vi "TestFastLocalizeCPULooped.vi"() -> ()   [LabVIEW 2011]
uses:
  CpuTrackDLL.vi
panel:
  out "Waveform Chart":sgl[](graph)
  in  "spotsize":sgl=20.0
  in  "ypos":sgl=128.0
  in  "xpos":sgl=128.0
  in  "Boolean":bool
  out "debug":T1(plugin-control)
  out "median":sgl
  out "xcorpos":cluster{"XCor X":sgl, "XCor Y":sgl}
  out "COM":cluster{"comX":sgl, "comY":sgl}
  out "Image":T1(plugin-control)
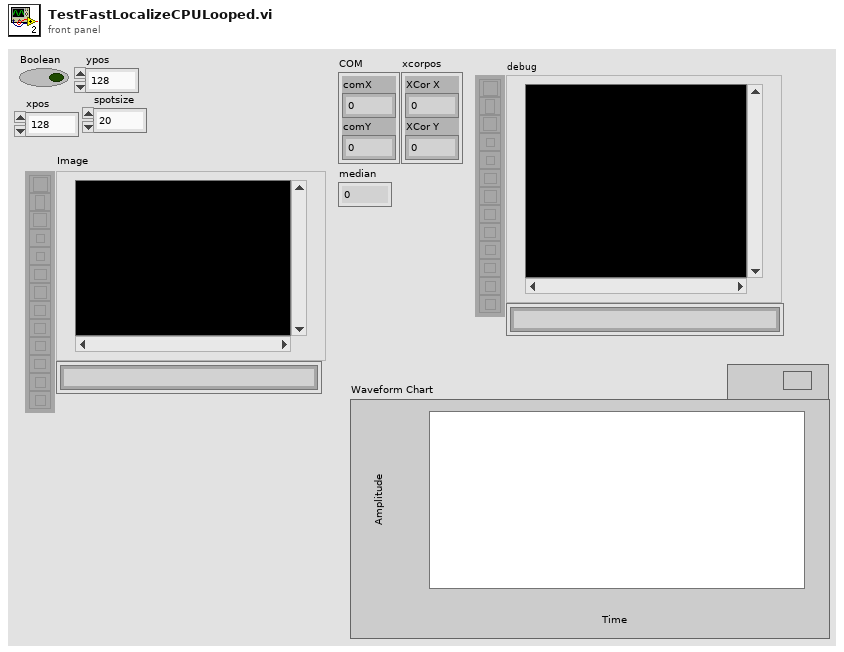
[diagram p1: front panel]
types:
  T1 = typedef "IMAQ Image.ctl" = refnum<image>
  T2 = typedef "Image Type" = u32
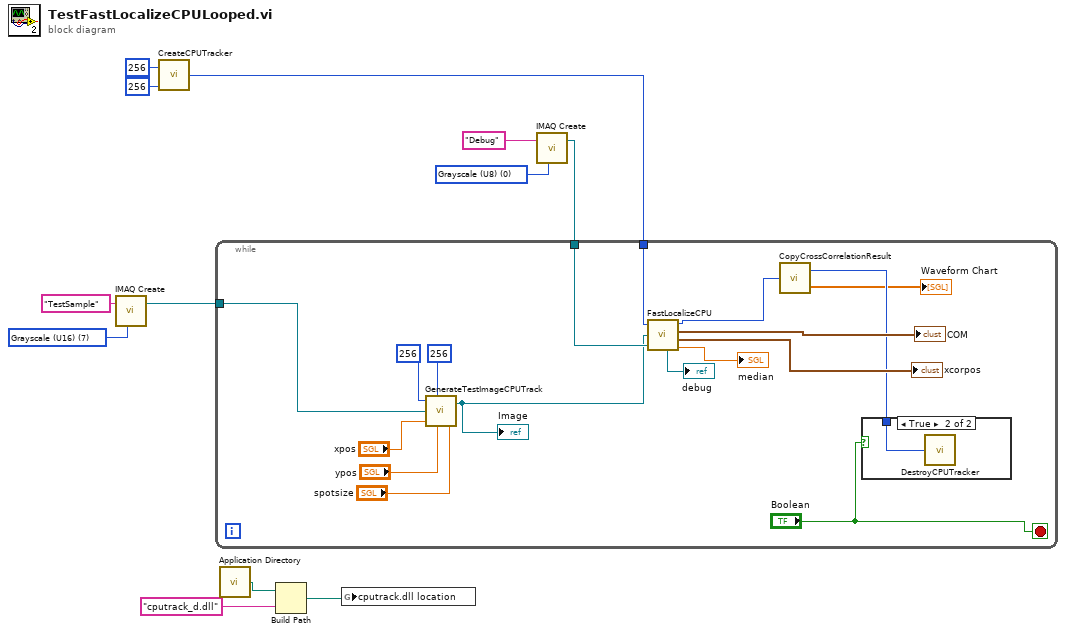
[diagram p0: block diagram]
diagram:
  w2 = T2 7 items=["Grayscale (U8)", "Grayscale (I16)", "Grayscale (SGL)", "Complex (CSG)", "RGB (U32)", "HSL (U32)", "RGB (U64)", "Grayscale (U16)"] ("Image Type")
  w11 = T2 0 items=["Grayscale (U8)", "Grayscale (I16)", "Grayscale (SGL)", "Complex (CSG)", "RGB (U32)", "HSL (U32)", "RGB (U64)", "Grayscale (U16)"] ("Image Type")
  n1 = call "IMAQ Create"("Image Name"="TestSample" ("String"), "Image Type"=w2) -> ("New Image"=w1:T1)  [unwired: 3 in, 1 out]
  n2 = call "CreateCPUTracker.vi"("height"=u32 256, "width"=u32 256) -> ("return type"=w4:u64)
  n3 = call <vilib>:"Application Directory.vi"() -> ("Application Directory"=w10:path)
  n4 = Build Path(base path=w10, name or relative path="cputrack_d.dll") -> (appended path=w8:path)
  n5 = global write "CpuTrackDLL.vi" "cputrack.dll location"(w8) -> ()
  n6 = call "IMAQ Create"("Image Name"="Debug" ("String"), "Image Type"=w11) -> ("New Image"=w5:T1)  [unwired: 3 in, 1 out]
  n7 = while {
    tunnel: w5 -> [w29]
    tunnel: w4 -> [w28]
    tunnel: w1 -> [w19]
    stop <- "Boolean" stop-if-true
    n8 = call "GenerateTestImageCPUTrack.vi"("width"=u32 256, "height"=u32 256, "image"=w19, "xpos"="xpos", "ypos"="ypos", "spotsize"="spotsize") -> ("Image"=w17:T1)
    "Image" <- w17
    n9 = call "FastLocalizeCPU.vi"("tracker"=w28, "input image"=w17, "debug image"=w29) -> ("tracker"=w15:u64, "COM"=→"COM":cluster{"comX":sgl, "comY":sgl}, "debug image"=→"debug":T1, "xcorpos"=→"xcorpos":cluster{"XCor X":sgl, "XCor Y":sgl}, "median"=→"median":sgl)  [unwired: 3 in]
    n10 = call "CopyCrossCorrelationResult.vi"("tracker"=w15) -> ("tracker"=w14:u64, "resultArray"=→"Waveform Chart":sgl[])
    n11 = case shown="True" "Boolean" {
      tunnel: w14 -> [_ w30]
      frame False {
      }
      frame True {
        n12 = call "DestroyCPUTracker.vi"("tracker"=w30) -> ()
      }
    }
  }
